vi "globales.vi"() -> ()   [LabVIEW 2019]
panel:
  in  "last_id_ajuste_previo":i32
  in  "Sim":bool
  in  "Vguardado":dbl
  in  "tipo_generador":string
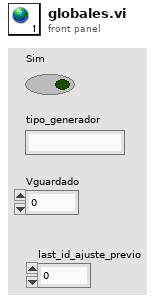
[diagram p1: front panel]
diagram:
